vi "Save Sweep Data to csv_kENA.vi"(4 "Meas Type":string="QuickView_", 5 "Selected Exp Settings":T13={"Floor_Sweep_Stop_V"=36.0, "Resistance Threshold"=1.0, "Floor_Sweep_Start_V"=36.0, "Floor_Sweep_Step_V"=1.0, "Roof_Sweep_Stop_V"=36.0, "Roof_Sweep_Start_V"=36.0, "Roof_Sweep_Step_V"=1.0, "Meas Type"=enum."Floor", "Experiment Name"=""}, 6 "Additional Data":T14, 7 "Filepath":path, 8 "Parametric Calculated Values":T5={"Voltage Calculated Values"={"P1_VPD_C"=0.0, "P2_VPD_C"=0.0, "P1_VPD_Rel_C"=0.0, "P2_VPD_Rel_C"=0.0}, "Resistance Calculated Values"={"Rc_free"=0.0, "Rc_first"=0.0, "Rc_vmax"=0.0, "Rc_last"=0.0, "Rc_end"=0.0, "VPD_R"=0.0, "VPD_Rel_R"=0.0}, "Capacitance Calculated Values"={"P1_CPD_free"=0.0, "P2_CPD_free"=0.0, "P1_CPD_vmax"=0.0, "P2_CPD_vmax"=0.0, "P1_CPD_first"=0.0, "P2_CPD_first"=0.0, "P1_CPD_last"=0.0, "P2_CPD_last"=0.0, "P1_CPD_end"=0.0, "P2_CPD_end"=0.0, "P1_CPD_max"=0.0, "P2_CPD_max "=0.0, "CPD_Free"=0.0, "CPD_First"=0.0, "CPD_max"=0.0, "CPD_Last"=0.0, "CPD_End"=0.0, "CPD_vmax"=0.0}, "Cap Calc Arrays"={"CPD_sum"=[], "P2_CPD@V"=[], "P1_CPD@V"=[], "Specific Voltages"=[32.0, 36.0]}, "Resistance Array Calc"={"RC@V"=[]}, "TN4 Calc"={"P1_TN4_ACT"=0.0, "P2_TN4_ACT "=0.0, "VPD_R_2"=0.0, "DVR"=0.0}, "Corrected_Capacitance Calculated Values"={"P1_CPD_free"=0.0, "P2_CPD_free"=0.0, "P1_CPD_vmax"=0.0, "P2_CPD_vmax"=0.0, "P1_CPD_first"=0.0, "P2_CPD_first"=0.0, "P1_CPD_last"=0.0, "P2_CPD_last"=0.0, "P1_CPD_end"=0.0, "P2_CPD_end"=0.0, "P1_CPD_max"=0.0, "P2_CPD_max "=0.0, "CPD_Free"=0.0, "CPD_First"=0.0, "CPD_max"=0.0, "CPD_Last"=0.0, "CPD_End"=0.0, "CPD_vmax"=0.0}}, 9 "ks5080A_Meaurements":T4, 10 "Date Cluster":T3, 11 "Test Information":T2={"Exp Name"="Cold Switching", "Lot"="0233A", "Wafer"="15", "Die Type"="L22", "Die X "="6", "Die Y"="8", "Exp"="1", "Die X_Y"="8"}) -> ()   [LabVIEW 2013]
uses:
  Controls/Date Control.ctl
  Controls/Test Information.ctl
  Controls/Parametric Calculated Values.ctl
  Controls/Voltage Calculated Values.ctl
  Controls/Resistance Individual Calculated Values.ctl
  Controls/Capacitance Individual Calculated Values.ctl
  Controls/Capacitance Array Calculated Values.ctl
  Controls/Resistance Array Calculated Values.ctl
  Controls/TN4 Calc.ctl
  Controls/Corrected_Capacitance Individual Calculated Values.ctl
  Controls/Additional Data.ctl
  Controls/ks5080A_Measurements.ctl
  Controls/Individual User Inputs_Floor and Roof.ctl
  <vilib>/Utility/file.llb/Write To Spreadsheet File (string).vi
panel:
  in  "Tab Control":T1(tab)
  # "Test Settings"
  # "Calculation Settings"
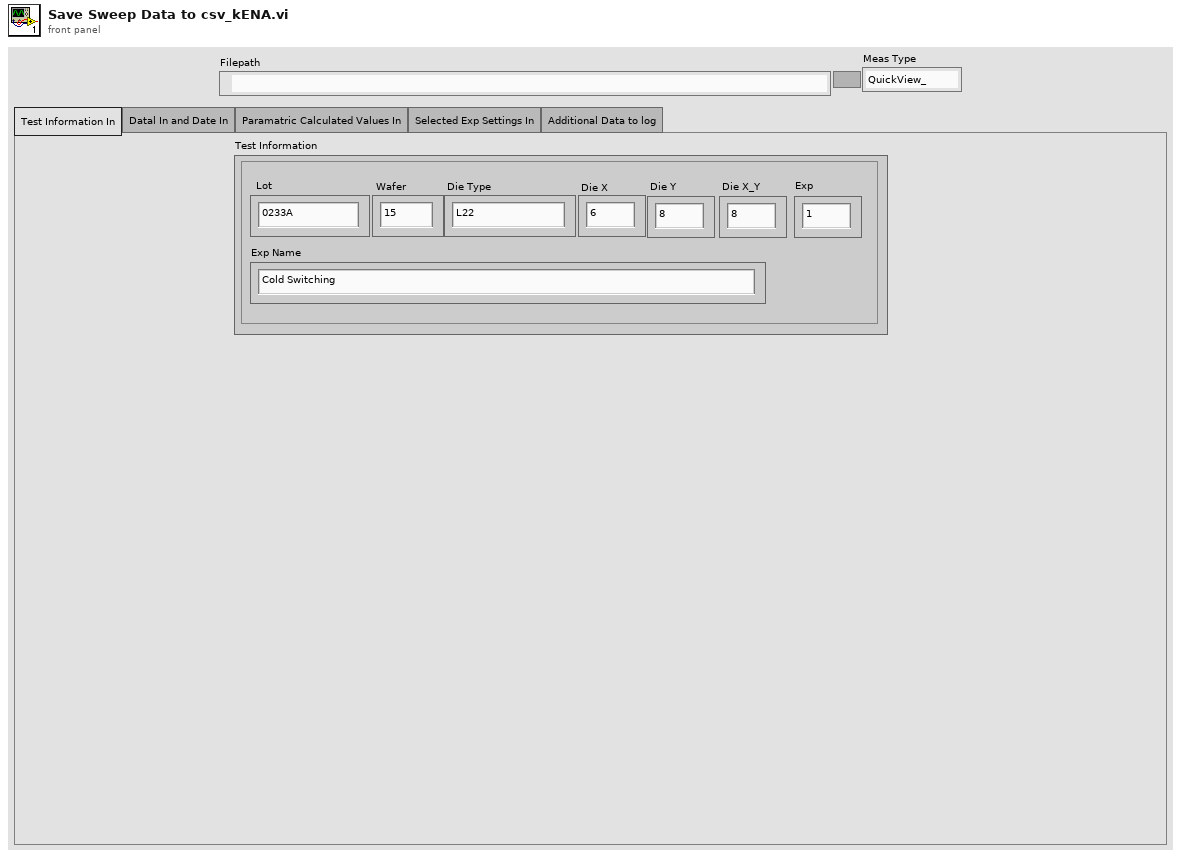
[diagram p1: front panel]
types:
  T1 = enum32{"Test Information In", "Datal In and Date In", "Paramatric Calculated Values In", "Selected Exp Settings In", "Additional Data to log"}
  T2 = typedef "Test Information.ctl" = cluster{"Exp Name":string, "Lot":string, "Wafer":string, "Die Type":string, "Die X ":string, "Die Y":string, "Exp":string, "Die X_Y":string}
  T3 = typedef "Date Control.ctl" = cluster{"Date":string, "Start Time":string, "Stop Time":string}
  T4 = typedef "ks5080A_Measurements.ctl" = cluster{"Bias_Sweep_Setting":dbl[], "Bias_voltage measurements":dbl[], "Bias_current measurements":dbl[], "P1_Capacitance":dbl[], "P2_Capacitance":dbl[], "DMM_Measurement_V":dbl[], "Contact_Source Current measurements":dbl[], "Contact_Sink Current measurements":dbl[], "Calculated_Resistance":dbl[], "P3_Capacitance":dbl[], "Port 1_S_parm":string[], "Port 2_S_parm":string[], "Port 3_S_parm":string[]}
  T5 = typedef "Parametric Calculated Values.ctl" = cluster{"Voltage Calculated Values":T6, "Resistance Calculated Values":T7, "Capacitance Calculated Values":T8, "Cap Calc Arrays":T9, "Resistance Array Calc":T10, "TN4 Calc":T11, "Corrected_Capacitance Calculated Values":T12}
  T6 = typedef "Voltage Calculated Values.ctl" = cluster{"P1_VPD_C":dbl, "P2_VPD_C":dbl, "P1_VPD_Rel_C":dbl, "P2_VPD_Rel_C":dbl}
  T7 = typedef "Resistance Individual Calculated Values.ctl" = cluster{"Rc_free":dbl, "Rc_first":dbl, "Rc_vmax":dbl, "Rc_last":dbl, "Rc_end":dbl, "VPD_R":dbl, "VPD_Rel_R":dbl}
  T8 = typedef "Capacitance Individual Calculated Values.ctl" = cluster{"P1_CPD_free":dbl, "P2_CPD_free":dbl, "P1_CPD_vmax":dbl, "P2_CPD_vmax":dbl, "P1_CPD_first":dbl, "P2_CPD_first":dbl, "P1_CPD_last":dbl, "P2_CPD_last":dbl, "P1_CPD_end":dbl, "P2_CPD_end":dbl, "P1_CPD_max":dbl, "P2_CPD_max ":dbl, "CPD_Free":dbl, "CPD_First":dbl, "CPD_max":dbl, "CPD_Last":dbl, "CPD_End":dbl, "CPD_vmax":dbl}
  T9 = typedef "Capacitance Array Calculated Values.ctl" = cluster{"CPD_sum":dbl[], "P2_CPD@V":dbl[], "P1_CPD@V":dbl[], "Specific Voltages":dbl[]}
  T10 = typedef "Resistance Array Calculated Values.ctl" = cluster{"RC@V":dbl[]}
  T11 = typedef "TN4 Calc.ctl" = cluster{"P1_TN4_ACT":dbl, "P2_TN4_ACT ":dbl, "VPD_R_2":dbl, "DVR":dbl}
  T12 = typedef "Corrected_Capacitance Individual Calculated Values.ctl" = cluster{"P1_CPD_free":dbl, "P2_CPD_free":dbl, "P1_CPD_vmax":dbl, "P2_CPD_vmax":dbl, "P1_CPD_first":dbl, "P2_CPD_first":dbl, "P1_CPD_last":dbl, "P2_CPD_last":dbl, "P1_CPD_end":dbl, "P2_CPD_end":dbl, "P1_CPD_max":dbl, "P2_CPD_max ":dbl, "CPD_Free":dbl, "CPD_First":dbl, "CPD_max":dbl, "CPD_Last":dbl, "CPD_End":dbl, "CPD_vmax":dbl}
  T13 = typedef "Individual User Inputs_Floor and Roof.ctl" = cluster{"Floor_Sweep_Stop_V":dbl, "Resistance Threshold":dbl, "Floor_Sweep_Start_V":dbl, "Floor_Sweep_Step_V":dbl, "Roof_Sweep_Stop_V":dbl, "Roof_Sweep_Start_V":dbl, "Roof_Sweep_Step_V":dbl, "Meas Type":enum16{"Floor", "Roof", "Floor and Roof"}, "Experiment Name":string}
  T14 = typedef "Additional Data.ctl" = cluster{"P2_Capacitance_PostTest":dbl[], "P1_Capacitance _PostTest":dbl[], "P1_Capacitance_PreTest":dbl[], "P2_Capacitance_PreTest":dbl[]}
  T15 = enum16{"open", "replace", "create", "open or create", "replace or create", "replace or create with confirmation"}
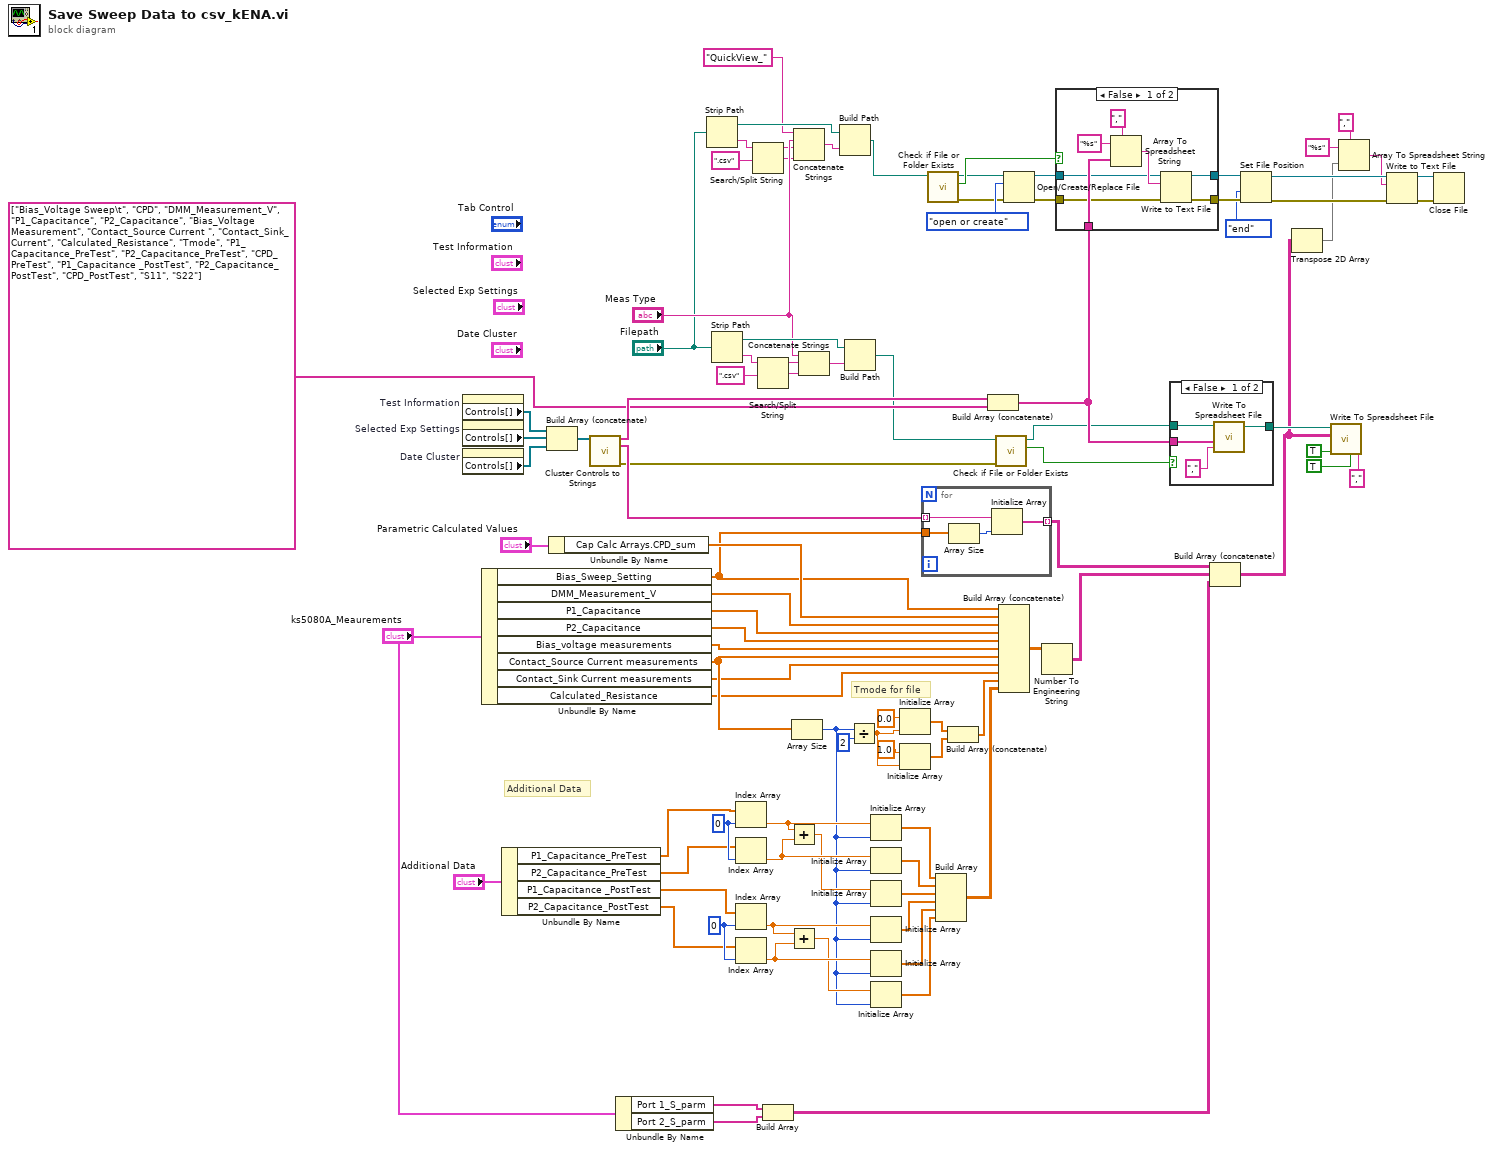
[diagram p0: block diagram]
diagram:
  w69 = 0 ("index")
  w70 = 0 ("index")
  # "Additional Data"
  # "Tmode for file"
  n1 = property on="Test Information" class="Clust (strict)"() -> ("Controls[]"=w95:refnum<vi>[])  [unwired: 2 in, 2 out]
  n2 = property on="Selected Exp Settings" class="Clust (strict)"() -> ("Controls[]"=w1:refnum<vi>[])  [unwired: 2 in, 2 out]
  n3 = property on="Date Cluster" class="Clust (strict)"() -> ("Controls[]"=w93:refnum<vi>[])  [unwired: 2 in, 2 out]
  n4 = Unbundle By Name("ks5080A_Meaurements") -> ("Bias_Sweep_Setting"=w43:dbl[], "DMM_Measurement_V"=w42:dbl[], "P1_Capacitance"=w41:dbl[], "P2_Capacitance"=w40:dbl[], "Bias_voltage measurements"=w39:dbl[], "Contact_Source Current measurements"=w38:dbl[], "Contact_Sink Current measurements"=w37:dbl[], "Calculated_Resistance"=w36:dbl[])
  n5 = Unbundle By Name("Additional Data") -> ("P1_Capacitance_PreTest"=w53:dbl[], "P2_Capacitance_PreTest"=w52:dbl[], "P1_Capacitance _PostTest"=w51:dbl[], "P2_Capacitance_PostTest"=w50:dbl[])
  n6 = Build Array (concatenate)(w95, w1, w93) -> (w94:refnum<vi>[])
  n7 = Unbundle By Name("Parametric Calculated Values") -> ("Cap Calc Arrays.CPD_sum"=w75:dbl[])
  n8 = call "Cluster Controls to Strings.vi"("Controls[]"=w94) -> ("Control Labels"=w78:string[], "Control Values"=w92:string[], "Error Out"=w77:errorcluster)  [unwired: 12 in]
  n9 = Unbundle By Name("ks5080A_Meaurements") -> ("Port 1_S_parm"=w34:string[], "Port 2_S_parm"=w33:string[])
  n10 = Strip Path(path="Filepath") -> (stripped path=w22:path, name=w25:string)
  n11 = Strip Path(path="Filepath") -> (stripped path=w46:path, name=w49:string)
  n12 = Index Array(array=w53, index=w70) -> (element=w68:dbl)
  n13 = Index Array(array=w52, index=w70) -> (element=w67:dbl)
  n14 = Index Array(array=w51, index=w69) -> (element=w65:dbl)
  n15 = Index Array(array=w50, index=w69) -> (element=w64:dbl)
  n16 = Search/Split String(string=w25, search string/char (-)=".csv" ("search string")) -> (substring before match=w20:string, match + rest of string=w23:string)  [unwired: 1 in, 1 out]
  n17 = Search/Split String(string=w49, search string/char (-)=".csv" ("search string")) -> (substring before match=w44:string, match + rest of string=w47:string)  [unwired: 1 in, 1 out]
  n18 = Build Array(w34, w33) -> (w32:string[][])
  n19 = Add(x=w68, y=w67) -> (x+y=w66:dbl)
  n20 = Add(x=w65, y=w64) -> (x+y=w63:dbl)
  n21 = Array Size(array=w38) -> (size(s)=w62:i32)
  n22 = Concatenate Strings("QuickView_" ("search string"), "Meas Type", w20, w23) -> (w21:string)
  n23 = Concatenate Strings("Meas Type", w44, w47) -> (w45:string)
  n24 = Build Path(base path=w22, name or relative path=w21) -> (appended path=w5:path)
  n25 = Build Path(base path=w46, name or relative path=w45) -> (appended path=w28:path)
  n26 = Divide(x=w62, y=2) -> (x/y=w90:dbl)
  n27 = Initialize Array(w68, w62) -> (w61:dbl[])
  n28 = Initialize Array(w67, w62) -> (w60:dbl[])
  n29 = Initialize Array(w66, w62) -> (w59:dbl[])
  n30 = Initialize Array(w65, w62) -> (w58:dbl[])
  n31 = Initialize Array(w64, w62) -> (w57:dbl[])
  n32 = Initialize Array(w63, w62) -> (w56:dbl[])
  n33 = Initialize Array(0.0, w90) -> (w91:dbl[])
  n34 = Initialize Array(1.0, w90) -> (w86:dbl[])
  n35 = for {
    tunnel: w43 -> [w99]
    tunnel: w92 -> [w98] mode=indexing
    tunnel: [w96] -> w81 mode=indexing
    n36 = Array Size(array=w99) -> (size(s)=w97:i32)
    n37 = Initialize Array(w98, w97) -> (w96:string[])
  }
  n38 = call <vilib>:"Check if File or Folder Exists.vi"("path"=w5) -> ("error out"=w4:errorcluster, "file or folder exists?"=w3:bool, "dup path"=w2:path)  [unwired: 8 in]
  n39 = Build Array(w61, w60, w59, w58, w57, w56) -> (w55:dbl[][])
  n40 = Build Array (concatenate)(w91, w86) -> (w71:dbl[])
  n41 = Build Array (concatenate)(w78, string[] ["Bias_Voltage Sweep\t", "CPD", "DMM_Measurement_V", "P1_Capacitance", "P2_Capacitance", "Bias_Voltage Measurement", "Contact_Source Current ", "Contact_Sink_Current", "Calculated_Resistance", "Tmode", "P1_Capacitance_PreTest", "P2_Capacitance_PreTest", "CPD_PreTest", "P1_Capacitance _PostTest", "P2_Capacitance_PostTest", "CPD_PostTest", "S11", "S22"]) -> (w73:string[])
  n42 = call <vilib>:"Check if File or Folder Exists.vi"("error in (no error)"=w77, "path"=w28) -> ("file or folder exists?"=w74:bool, "dup path"=w27:path)  [unwired: 7 in, 1 out]
  n43 = Build Array (concatenate)(w43, w75, w42, w41, w40, w39, w38, w37, w36, w71, w55) -> (w79:dbl[][])
  n44 = Open/Create/Replace File(file path (use dialog)=w2, error in=w4, operation (0:open)=T15."open or create") -> (refnum out=w19:refnum<file>, error out=w18:errorcluster)  [unwired: 3 in, 1 out]
  n45 = Number To Engineering String(4:w79) -> (0:w80:string[][])  [unwired: 3 in]
  n46 = case shown="False" w3 {
    tunnel: w73 -> [w105 _]
    tunnel: w19 -> [w103 w109]
    tunnel: w18 -> [w102 w108]
    tunnel: [w101 w108] -> w16
    tunnel: [w100 w109] -> w17
    frame False {
      n47 = Array To Spreadsheet String(delimiter (Tab)="," ("delimiter (\\t)"), array=w105, 3:"%s" ("format string")) -> (spreadsheet string=w104:string)
      n48 = Write to Text File(file (use dialog)=w103, text=w104, error in=w102) -> (refnum out=w100:refnum<file>, error out=w101:errorcluster)  [unwired: 1 in, 1 out]
    }
    frame True {
    }
  }
  n49 = case shown="False" w74 {
    tunnel: w27 -> [w113 w114]
    tunnel: w73 -> [w112 _]
    tunnel: [w110 w114] -> w85
    frame False {
      n50 = call-poly <vilib>:"Write To Spreadsheet File.vi"("delimiter (\\t)"="," ("delimiter (\\t)"), "1D data"=w112, "file path (dialog if empty)"=w113) -> ("new file path (Not A Path if cancelled)"=w110:path)  [unwired: 5 in]
    }
    frame True {
    }
  }
  n51 = Build Array (concatenate)(w81, w80, w32) -> (w72:string[][])
  n52 = Set File Position(refnum=w17, from (0:start)=enum16{"start", "end", "current"}."end", error in=w16) -> (refnum out=w11:refnum<file>, error out=w12:errorcluster)  [unwired: 1 in]
  n53 = Transpose 2D Array(2D array=w72) -> (transposed array=w7:string[][])
  n54 = call-poly <vilib>:"Write To Spreadsheet File.vi"("delimiter (\\t)"="," ("delimiter (\\t)"), "transpose? (no:F)"=TRUE, "append to file? (new file:F)"=TRUE, "2D data"=w72, "file path (dialog if empty)"=w85) -> ()  [unwired: 3 in, 1 out]
  n55 = Array To Spreadsheet String(delimiter (Tab)="," ("delimiter (\\t)"), array=w7, 3:"%s" ("format string")) -> (spreadsheet string=w10:string)
  n56 = Write to Text File(file (use dialog)=w11, text=w10, error in=w12) -> (refnum out=w8:refnum<file>, error out=w9:errorcluster)  [unwired: 1 in, 1 out]
  n57 = Close File(refnum=w8, error in=w9) -> ()  [unwired: 2 out]
